vi "parse settings set.vi"(1 "settings in":string) -> (0 "settings out":string[](array[string]))   [LabVIEW 2024, in "controls manager.lvlib"]
uses:
  controls manager.lvlib
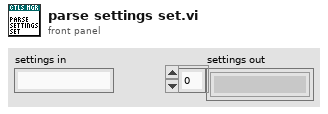
[diagram p1: front panel]
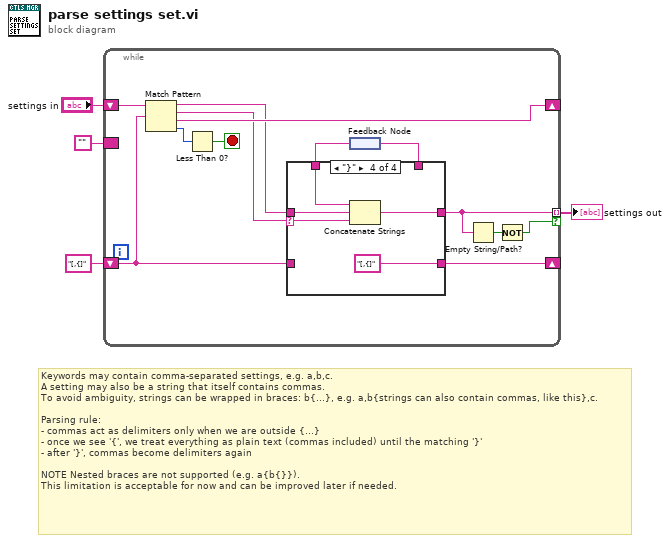
[diagram p0: block diagram]
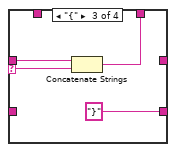
[diagram p4: hidden frame]
diagram:
  # "Keywords may contain comma-separated settings, e.g. a,b,c.\nA setting may also be a string that itself contains commas.\nTo avoid ambiguity, strings can be wrapped in braces: b{...}, e.g. a,b{strings can also contain commas, like this},c.\n\nParsing rule:\n- commas act as delimiters only when we are outside {...}\n- once we see '{', we treat everything as plain text (commas included) until the matching '}'\n- after '}', commas become delimiters again\n\nNOTE Nested braces are not supported (e.g. a{b{}}).\nThis limitation is acceptable for now and can be improved later if needed."
  n1 = while {
    tunnel: [w7] -> w2 mode=indexing if=w5
    shift-right: [w12] -> _
    shift-left: "[,{]" -> [w11]
    shift-right: [w17] -> _
    shift-left: "settings in" -> [w16]
    border: "" -> [_]
    stop <- w14 stop-if-true
    n2 = Match Pattern(string=w16, regular expression=w11) -> (before substring=w10:string, match substring=w13:string, after substring=w17:string, offset past match=w15:i32)  [unwired: 1 in]
    n3 = Less Than 0?(x=w15) -> (x < 0?=w14:bool)
    n4 = feedback #1() -> (w8:string)
    n5 = case shown="\"}\"" w13 {
      selector: w13 -> [_ _ w23 w27]
      tunnel: w10 -> [w19 w21 w24 w28]
      tunnel: [w19 w21 _ w26] -> w7
      tunnel: [w18 w20 "}" "[,{]"] -> w12
      tunnel: w11 -> [w18 w20 _ _]
      tunnel: [_ _ w22 _] -> w9
      tunnel: w8 -> [_ _ _ w29]
      frame Default {
      }
      frame "," {
      }
      frame "{" {
        n6 = Concatenate Strings(w24, w23) -> (w22:string)
      }
      frame "}" {
        n7 = Concatenate Strings(w29, w28, w27) -> (w26:string)
      }
    }
    n8 = feedback-in #1(w9) -> ()
    n9 = Empty String/Path?(string/path=w7) -> (empty?=w6:bool)
    n10 = Not(x=w6) -> (.not. x?=w5:bool)
  }
  "settings out" <- w2
